vi "预览结果显示.vi"(1 "预览结果":string) -> (0 "预览结果 2":string caption="预览结果")   [LabVIEW 2013]
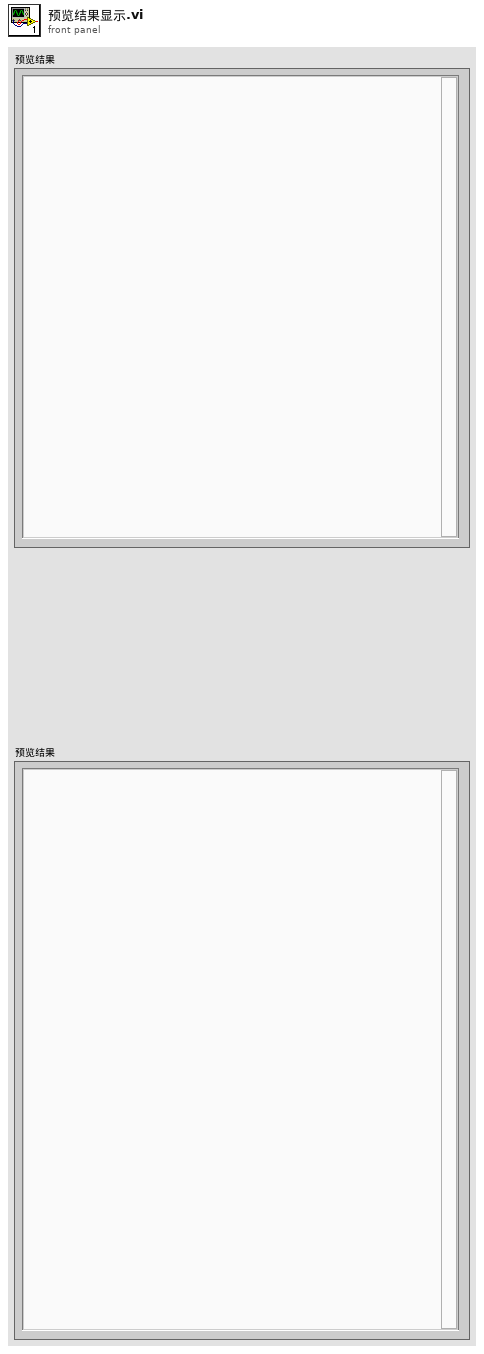
[diagram p1: front panel]
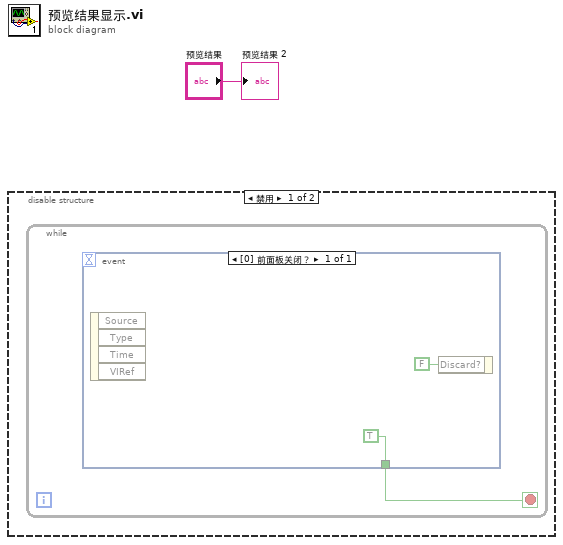
[diagram p0: block diagram]
diagram:
  n1 = disable-structure shown="禁用" {
    frame Disabled {
      n2 = while {
        stop <- w2 stop-if-true
        n3 = event shown="[0] 前面板关闭？" {
          selector: _ -> [_]
          dyn-events: _ -> [_]
          timeout: _ -> [_]
          tunnel: [TRUE] -> w2
          event Panel Close? {
            n4 = event-data() -> ()  [unwired: 1 in, 4 out]
            n5 = event-data("Discard?"=FALSE ("放弃？")) -> ()  [unwired: 1 in, 1 out]
          }
        }
      }
    }
    frame Enabled {
    }
  }
  "预览结果 2" <- "预览结果"
